vi "EncodeString.vi"(1 "string":string="TEST") -> (0 "Boolean array":bool[](array[boolean]))   [LabVIEW 2016]
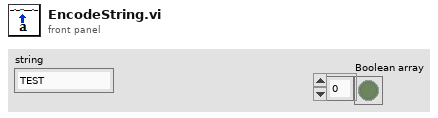
[diagram p1: front panel]
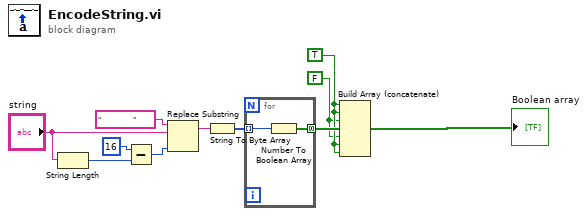
[diagram p0: block diagram]
diagram:
  w2 = FALSE
  w3 = TRUE
  n1 = String Length(string="string") -> (length=w10:i32)
  n2 = Subtract(x=16, y=w10) -> (x-y=w6:i32)
  n3 = Replace Substring(2:w6, 4:"string", 5:"                " ("string")) -> (1:w5:string)  [unwired: 1 in, 1 out]
  n4 = String To Byte Array(string=w5) -> (unsigned byte array=w11:u8[])
  n5 = for {
    tunnel: w11 -> [w13] mode=indexing
    tunnel: [w12] -> w4 mode=concatenating
    n6 = Number To Boolean Array(number=w13) -> (Boolean array=w12:bool[])
  }
  n7 = Build Array (concatenate)(w3, w3, w2, w4, w2, w3, w3) -> (→"Boolean array":bool[])
